vi "B07_Save_changed_PVs.vi"(5 "For Test":bool, 7 "想要限制的筆數":i32=1000, 8 "error in":errorcluster, 9 "Directory Path":path, 10 "紀錄起始時間  門檻":dbl=3591721451.0 format="%#_13g", 11 "diff_Value 2":string[][](array[string])=[["2017/10/25 04:24", "SR-DI-DCCT:BeamCurrent", "341.599", "341.619", "3591721448.059474"], ["2017/10/25 04:24", "SR-DI-DCCT:BeamCurrent", "341.587", "341.599", "3591721449.159196"], ["2017/10/25 04:24", "SR-DI-DCCT:BeamCurrent", "341.576", "341.587", "3591721450.259158"], ["2017/10/25 04:24", "SR-DI-DCCT:BeamCurrent", "341.563", "341.576", "3591721451.359663"], ["2017/10/25 04:24", "SR-DI-DCCT:BeamCurrent", "341.553", "341.563", "3591721452.458849"], ["2017/10/25 04:24", "SR-DI-DCCT:BeamCurrent", "341.537", "341.553", "3591721453.558763"], ["2017/10/25 04:24", "SR-DI-DCCT:BeamCurrent", "341.527", "341.537", "3591721454.659339"], ["2017/10/25 04:24", "SR-DI-DCCT:BeamCurrent", "341.508", "341.527", "3591721455.760254"], ["2017/10/25 04:24", "SR-DI-DCCT:BeamCurrent", "341.5", "341.508", "3591721456.859482"], ["2017/10/25 04:24", "SR-DI-DCCT:BeamCurrent", "341.488", "341.5", "3591721457.959021"]]) -> (0 "error out":errorcluster, 3 "saved file path":path)   [LabVIEW 2017]
panel:
  out "concatenated string":string
  out "diff_Value":string[][](array[string])=[["2017/10/25 04:24", "SR-DI-DCCT:BeamCurrent", "341.599", "341.619", "3591721448.059474"], ["2017/10/25 04:24", "SR-DI-DCCT:BeamCurrent", "341.587", "341.599", "3591721449.159196"], ["2017/10/25 04:24", "SR-DI-DCCT:BeamCurrent", "341.576", "341.587", "3591721450.259158"], ["2017/10/25 04:24", "SR-DI-DCCT:BeamCurrent", "341.563", "341.576", "3591721451.359663"], ["2017/10/25 04:24", "SR-DI-DCCT:BeamCurrent", "341.553", "341.563", "3591721452.458849"], ["2017/10/25 04:24", "SR-DI-DCCT:BeamCurrent", "341.537", "341.553", "3591721453.558763"], ["2017/10/25 04:24", "SR-DI-DCCT:BeamCurrent", "341.527", "341.537", "3591721454.659339"], ["2017/10/25 04:24", "SR-DI-DCCT:BeamCurrent", "341.508", "341.527", "3591721455.760254"], ["2017/10/25 04:24", "SR-DI-DCCT:BeamCurrent", "341.5", "341.508", "3591721456.859482"], ["2017/10/25 04:24", "SR-DI-DCCT:BeamCurrent", "341.488", "341.5", "3591721457.959021"]]
  out "subarray 2":string[][](array[string])=[["Time            ", "PV_name        ", "Ori_Value", "New_Value "], ["2017/10/25 04:24", "SR-DI-DCCT:BeamCurrent", "341.576", "341.587"], ["2017/10/25 04:24", "SR-DI-DCCT:BeamCurrent", "341.563", "341.576"], ["2017/10/25 04:24", "SR-DI-DCCT:BeamCurrent", "341.553", "341.563"], ["2017/10/25 04:24", "SR-DI-DCCT:BeamCurrent", "341.537", "341.553"], ["2017/10/25 04:24", "SR-DI-DCCT:BeamCurrent", "341.527", "341.537"], ["2017/10/25 04:24", "SR-DI-DCCT:BeamCurrent", "341.508", "341.527"], ["2017/10/25 04:24", "SR-DI-DCCT:BeamCurrent", "341.5", "341.508"], ["2017/10/25 04:24", "SR-DI-DCCT:BeamCurrent", "341.488", "341.5"]]
  out "size(s)":i32[](array[numeric])=[10, 5]
  out "LV_Time_DBL_format":string[](array[string])=["3591721448.059474", "3591721449.159196", "3591721450.259158", "3591721451.359663", "3591721452.458849", "3591721453.558763", "3591721454.659339", "3591721455.760254", "3591721456.859482", "3591721457.959021"]
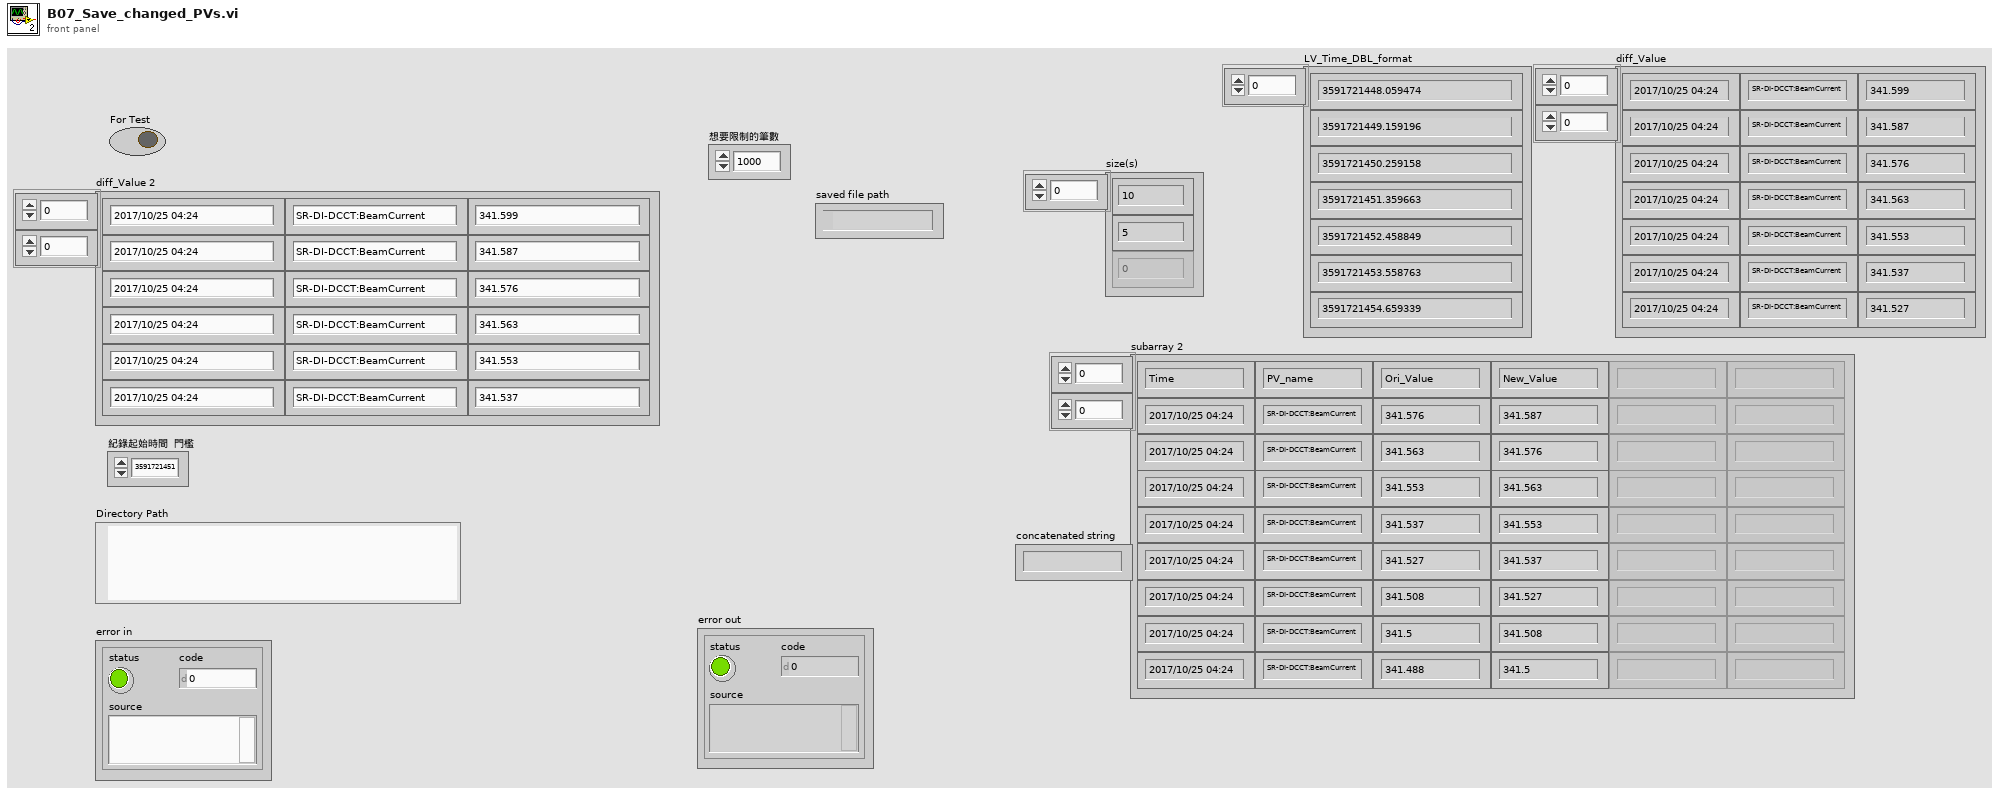
[diagram p1: front panel]
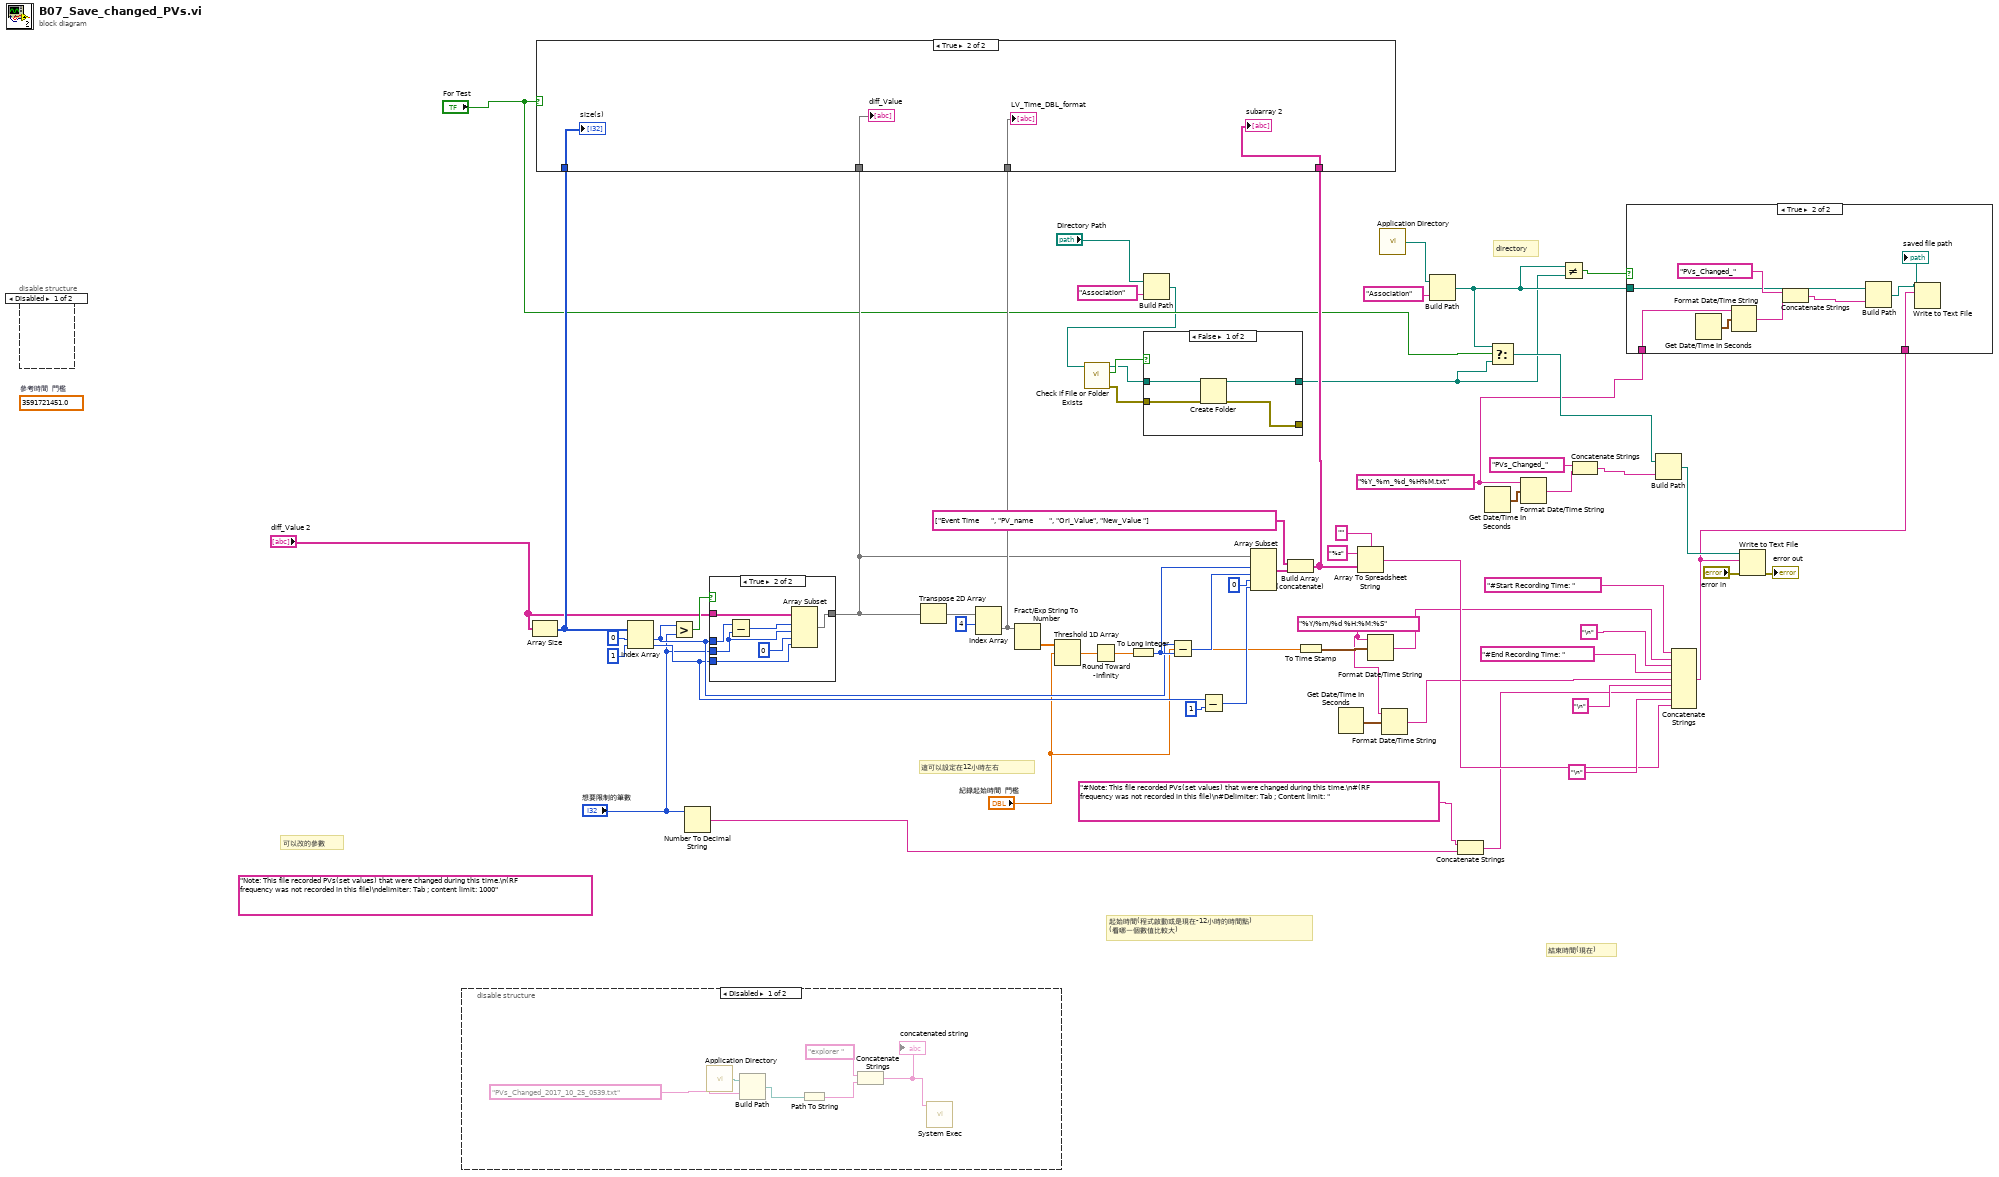
[diagram p0: block diagram]
diagram:
  w20 = "%Y/%m/%d %H:%M:%S" ("time format string (%c)")
  (unwired) "Note: This file recorded PVs(set values) that were changed during this time.\n(RF frequency was not recorded in this file)\ndelimiter: Tab ; content limit: 1000" ("time format string (%c)")
  w12 = "%Y_%m_%d_%H%M.txt" ("time format string (%c)")
  (unwired) 3591721451.0  # 參考時間  門檻
  # "directory"
  # "結束時間(現在)"
  # "起始時間(程式啟動或是現在-12小時的時間點)\n(看哪一個數值比較大)"
  # "可以改的參數"
  # "這可以設定在12小時左右"
  n1 = disable-structure shown="Disabled" {
    frame Disabled {
    }
    frame Enabled {
    }
  }
  n2 = disable-structure shown="Disabled" {
    frame Disabled {
      n3 = call <vilib>:"Application Directory.vi"() -> ("Application Directory"=w63:path)
      n4 = Build Path(base path=w63, name or relative path="PVs_Changed_2017_10_25_0539.txt") -> (appended path=w65:path)
      n5 = Path To String(path=w65) -> (string=w67:string)
      n6 = Concatenate Strings("explorer ", w67) -> (w68:string)
      "concatenated string" <- w68
      n7 = call <vilib>:"System Exec.vi"("command line"=w68) -> ()  [unwired: 7 in, 4 out]
    }
    frame Enabled {
    }
  }
  n8 = Array Size(array="diff_Value 2") -> (size(s)=w56:i32[])
  n9 = Index Array(array=w56, index #1=0 ("index"), index #2=1 ("index")) -> (element #1=w42:i32, element #2=w41:i32)
  n10 = Greater?(x=w42, y="想要限制的筆數") -> (0:w40:bool)
  n11 = Number To Decimal String(number="想要限制的筆數") -> (decimal integer string=w27:string)  [unwired: 1 in]
  n12 = case shown="True" w40 {
    tunnel: "diff_Value 2" -> [w69 w75]
    tunnel: w42 -> [_ w74]
    tunnel: "想要限制的筆數" -> [_ w73]
    tunnel: w41 -> [_ w71]
    tunnel: [w69 w70] -> w38
    frame False {
    }
    frame True {
      n13 = Subtract(x=w74, y=w73) -> (x-y=w72:i32)
      n14 = Array Subset(array=w75, index (row)=w72, length (row)=w73, index (col)=0 ("index"), length (col)=w71) -> (w70:string[][])
    }
  }
  n15 = Transpose 2D Array(2D array=w38) -> (transposed array=w61:string[][])
  n16 = Index Array(array=w61, index (row)=4) -> (element=w60:string[])  [unwired: 1 in]
  n17 = Fract/Exp String To Number(string=w60) -> (number=w59:dbl[])  [unwired: 3 in, 1 out]
  n18 = Threshold 1D Array(2:"紀錄起始時間  門檻", 3:w59) -> (0:w58:dbl)  [unwired: 1 in]
  n19 = Round Toward -Infinity(1:w58) -> (0:w57:dbl)
  n20 = To Long Integer(number=w57) -> (32bit integer=w52:i32)
  n21 = Build Path(base path="Directory Path", name or relative path="Association" ("string")) -> (appended path=w6:path)
  n22 = call <vilib>:"Check if File or Folder Exists.vi"("path"=w6) -> ("error out"=w9:errorcluster, "file or folder exists?"=w11:bool, "dup path"=w10:path)  [unwired: 8 in]
  n23 = case shown="False" w11 {
    tunnel: w10 -> [w80 w81]
    tunnel: [w79 w82] -> _
    tunnel: w9 -> [w78 w82]
    tunnel: [w77 w81] -> w2
    frame False {
      n24 = Create Folder(path (use dialog)=w80, error in=w78) -> (created path=w77:path, error out=w79:errorcluster)  [unwired: 1 in, 1 out]
    }
    frame True {
    }
  }
  n25 = Subtract(x=w42, y=w52) -> (x-y=w53:i32)
  n26 = Subtract(x=w41, y=1) -> (x-y=w45:i32)
  n27 = Array Subset(array=w38, index (row)=w52, length (row)=w53, index (col)=0 ("index"), length (col)=w45) -> (w43:string[][])
  n28 = Build Array (concatenate)(string[] ["Event Time      ", "PV_name        ", "Ori_Value", "New_Value "] ("diff_Value"), w43) -> (w16:string[][])
  n29 = case shown="True" "For Test" {
    tunnel: w60 -> [_ w86]
    tunnel: w56 -> [_ w85]
    tunnel: w38 -> [_ w84]
    tunnel: w16 -> [_ w83]
    frame False {
    }
    frame True {
      "LV_Time_DBL_format" <- w86
      "size(s)" <- w85
      "diff_Value" <- w84
      "subarray 2" <- w83
    }
  }
  n30 = To Time Stamp(1:"紀錄起始時間  門檻") -> (0:w23:timestamp)
  n31 = Get Date/Time In Seconds() -> (seconds since 1Jan1904=w21:timestamp)
  n32 = Array To Spreadsheet String(delimiter (Tab)="", array=w16, 3:"%s" ("format string")) -> (spreadsheet string=w29:string)
  n33 = Format Date/Time String(time format string (%c)=w20, seconds (now)=w23) -> (date/time string=w22:string)  [unwired: 1 in]
  n34 = call <vilib>:"Application Directory.vi"() -> ("Application Directory"=w4:path)
  n35 = Format Date/Time String(time format string (%c)=w20, seconds (now)=w21) -> (date/time string=w19:string)  [unwired: 1 in]
  n36 = Build Path(base path=w4, name or relative path="Association" ("string")) -> (appended path=w3:path)
  n37 = Concatenate Strings("#Note: This file recorded PVs(set values) that were changed during this time.\n#(RF frequency was not recorded in this file)\n#Delimiter: Tab ; Content limit: " ("time format string (%c)"), w27) -> (w25:string)
  n38 = Get Date/Time In Seconds() -> (seconds since 1Jan1904=w50:timestamp)
  n39 = Select(t=w3, s="For Test", f=w2) -> (s? t:f=w14:path)
  n40 = Format Date/Time String(time format string (%c)=w12, seconds (now)=w50) -> (date/time string=w31:string)  [unwired: 1 in]
  n41 = Not Equal?(x=w3, y=w2) -> (x != y?=w1:bool)
  n42 = Concatenate Strings("PVs_Changed_" ("string"), w31) -> (w30:string)
  n43 = Build Path(base path=w14, name or relative path=w30) -> (appended path=w47:path)
  n44 = Concatenate Strings("#Start Recording Time: " ("time format string (%c)"), w22, "\n" ("time format string (%c)"), "#End Recording Time: " ("time format string (%c)"), w19, "\n" ("time format string (%c)"), w25, "\n" ("time format string (%c)"), w29) -> (w13:string)
  n45 = case shown="True" w1 {
    tunnel: w13 -> [_ w89]
    tunnel: w12 -> [_ w88]
    tunnel: w3 -> [_ w87]
    frame False {
    }
    frame True {
      n46 = Get Date/Time In Seconds() -> (seconds since 1Jan1904=w91:timestamp)
      n47 = Format Date/Time String(time format string (%c)=w88, seconds (now)=w91) -> (date/time string=w93:string)  [unwired: 1 in]
      n48 = Concatenate Strings("PVs_Changed_" ("string"), w93) -> (w94:string)
      n49 = Build Path(base path=w87, name or relative path=w94) -> (appended path=w90:path)
      "saved file path" <- w90
      n50 = Write to Text File(file (use dialog)=w90, text=w89) -> ()  [unwired: 2 in, 3 out]
    }
  }
  n51 = Write to Text File(file (use dialog)=w47, text=w13, error in="error in") -> (error out=→"error out":errorcluster)  [unwired: 1 in, 2 out]
